vi "XIPIN_AXI_Timer_2_0.vi"   [LabVIEW 2017]
doc: "The AXI Timer/Counter is a 32/64-bit timer module that attaches to the AXI4-Lite interface\n------------------------------------\n<b>Need License</b> : No\n<b>Interface</b> : AXI4"
uses:
  <vilib>/rvi/XilinxIP/XIPIN_XNode/niFpgaXIPIN.xnode
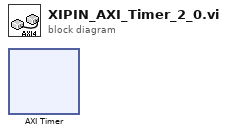
[diagram p0: block diagram]
diagram:
  n1 = xnode ("AXI Timer")() -> ()
